vi "Signal Conditioning (SubVI).vi"(11 "Input":dbl) -> (3 "Output":dbl)   [LabVIEW 2016]
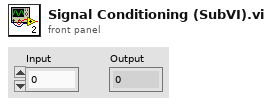
[diagram p1: front panel]
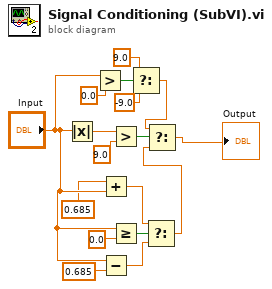
[diagram p0: block diagram]
diagram:
  n1 = Absolute Value(x="Input") -> (abs(x)=w7:dbl)
  n2 = Greater?(x="Input", y=0.0) -> (0:w13:bool)
  n3 = Add(x=0.685, y="Input") -> (x+y=w5:dbl)
  n4 = Subtract(x="Input", y=0.685) -> (x-y=w6:dbl)
  n5 = Greater?(x=w7, y=9.0) -> (0:w9:bool)
  n6 = Greater Or Equal?(x="Input", y=0.0) -> (x >= y?=w4:bool)
  n7 = Select(t=9.0, s=w13, f=-9.0) -> (s? t:f=w16:dbl)
  n8 = Select(t=w5, s=w4, f=w6) -> (s? t:f=w10:dbl)
  n9 = Select(t=w16, s=w9, f=w10) -> (s? t:f=→"Output":dbl)
